vi "WaveformBufferGeneration_(multi).vi"(5 "Amplitude":dbl=2.0 format="%0.2p", 6 "Cycles per Buffer":dbl=1.0 format="%.2f", 7 "Samples per Buffer":dbl=1000.0, 8 "error in (no error)":errorcluster, 9 "Waveform Type":T1(ring), 10 "Desired Frequency":dbl=1000.0 format="%.2f", 11 "task/channels in":refnum<k21>) -> (0 "error out":errorcluster, 1 "Resulting Frequency":dbl format="%.2f", 2 "Waveform":waveform(dbl)[](array[waveform]), 3 "task out":refnum<k21>, 4 "Resulting Sample Clock Rate":dbl format="%.2f")   [LabVIEW 2011]
doc: "This subVI is used to create a Sine, Square, Triangle or Sawtooth Waveform. The inputs to this VI are the Waveform Type, which determines if the output waveform is a Sine, Square, Triangle, or Sawtooth Waveform, the amplitude, Desired Frequency, Samples per Buffer, and Cycles per Buffer. \n\nThe Desired Frequency, Samples per Buffer, and Cycles per Buffer are used to calculate the sample clock rate. The DAQmx Timing property node sets the sample clock rate for the device specified in the task/channels in control. \n\nThe actual, coerced, sample clock rate is returned and used as an input to the Basic Function Generator.vi. The Basic Function Generator returns a waveform of data with timing information.\n\nThe formula below was used to determine the sample clock rate:\n\nDesired Frequency=[(Cycles/Buffer)X(Sample Clock Rate)]/Samples per Buffer\n\nNote: The Block Diagram rearranges the variables to solve for Sample Clock Rate"
uses:
  <vilib>/measure/NI_MABase.lvlib
  Program Files/National Instruments/LabVIEW 2011/resource/objmgr/daqmx.rc
panel:
  out "Samples/cycle":dbl format="%0.2f"
  out "Desired Sample Clock Rate":dbl format="%.2f"
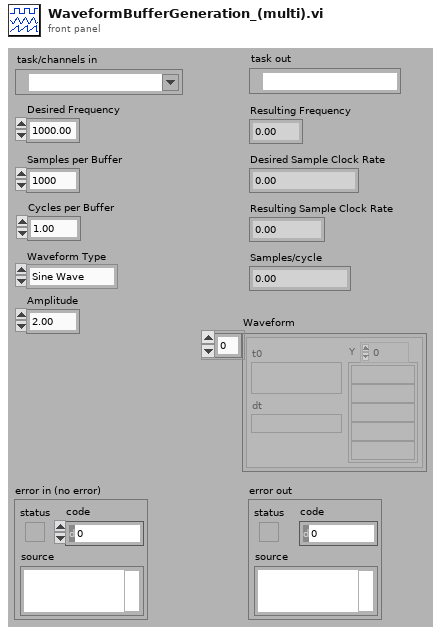
[diagram p1: front panel]
types:
  T1 = enum16{"Sine Wave", "Triangle Wave", "Square Wave", "Sawtooth Wave"}
  T2 = cluster{"SampClk.Rate":dbl, "Samples per Buffer":dbl}
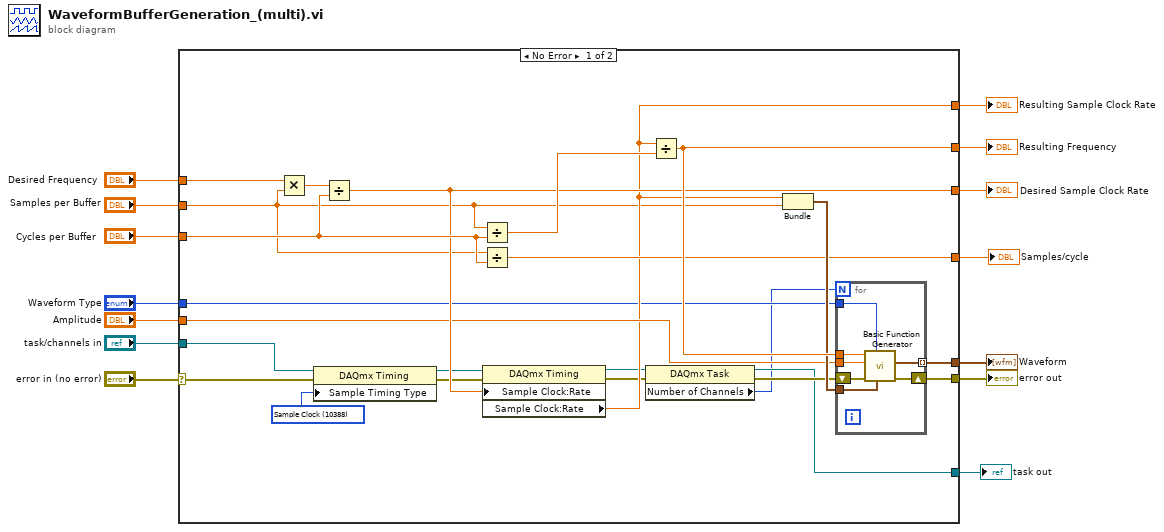
[diagram p0: block diagram]
diagram:
  n1 = case shown="No Error" "error in (no error)" {
    selector: "error in (no error)" -> [w16 w46]
    tunnel: [w38 _] -> w14
    tunnel: "Desired Frequency" -> [w37 _]
    tunnel: [w34 _] -> w12
    tunnel: "Cycles per Buffer" -> [w33 _]
    tunnel: [w31 _] -> w10
    tunnel: "Amplitude" -> [w30 _]
    tunnel: "Samples per Buffer" -> [w15 _]
    tunnel: [w29 _] -> w7
    tunnel: [w28 w46] -> w6
    tunnel: "task/channels in" -> [w24 _]
    tunnel: [w20 _] -> w4
    tunnel: [w19 _] -> w3
    tunnel: "Waveform Type" -> [w18 _]
    frame No Error {
      w25 = 10388 items=["Sample Clock"=10388, "Handshake"=10389, "Implicit"=10451, "On Demand"=10390, "Change Detection"=12504] ("SampTimingType")
      n2 = Multiply(x=w37, y=w15) -> (x*y=w35:dbl)
      n3 = property class="DAQmx Timing"(reference=w24, error in=w16, "Sample Timing Type"=w25) -> (reference out=w27:refnum<k21>, error out=w26:errorcluster)
      n4 = Divide(x=w35, y=w33) -> (x/y=w31:dbl)
      n5 = Divide(x=w15, y=w33) -> (x/y=w32:dbl)
      n6 = Divide(x=w15, y=w33) -> (x/y=w34:dbl)
      n7 = property class="DAQmx Timing"(reference=w27, error in=w26, "Sample Clock:Rate"=w31) -> (reference out=w22:refnum<k21>, error out=w23:errorcluster, "Sample Clock:Rate"=w29:dbl)
      n8 = property class="DAQmx Task"(reference=w22, error in=w23) -> (reference out=w20:refnum<k21>, error out=w21:errorcluster, "Number of Channels"=w17:u32)
      n9 = Divide(x=w29, y=w32) -> (x/y=w38:dbl)
      n10 = Bundle("SampClk.Rate"=w29, "Samples per Buffer"=w15) -> (w36:T2)  [unwired: 1 in]
      n11 = for {
        N: w17 -> [_]
        tunnel: w38 -> [w45]
        tunnel: w36 -> [w44]
        tunnel: [w43] -> w19 mode=indexing
        tunnel: w30 -> [w42]
        shift-right: [w41] -> w28
        shift-left: w21 -> [w40]
        tunnel: w18 -> [w39]
        n12 = call <vilib>:"Basic Function Generator.vi"("sampling info"=w44, "signal type"=w39, "error in (no error)"=w40, "amplitude"=w42, "frequency"=w45) -> ("error out"=w41:errorcluster, "signal out"=w43:waveform(dbl))  [unwired: 4 in, 1 out]
      }
    }
    frame Error {
    }
  }
  "Resulting Sample Clock Rate" <- w7
  "Desired Sample Clock Rate" <- w10
  "Resulting Frequency" <- w14
  "Samples/cycle" <- w12
  "error out" <- w6
  "task out" <- w4
  "Waveform" <- w3
